vi "COB send.vi"(4 "Data":u8[](array[numeric]), 5 "error in (no error)":errorcluster, 7 "COB id":i32) -> (0 "error out":errorcluster)   [LabVIEW 2023, in "canopen.lvlib" / "CANopen.lvclass"]
doc: "Sends a bunch of data to a specific COB-ID."
uses:
  CANopen.lvclass
  <vilib>/xnet/xnet.llb/XNET Frame CAN.ctl
  <vilib>/xnet/xnet.llb/XNET Frame Type CAN.ctl
  <vilib>/xnet/xnet.llb/XNET Write (Frame CAN).vi
panel:
  out "session out":refnum<k21>
  in  "session in":refnum<k21>
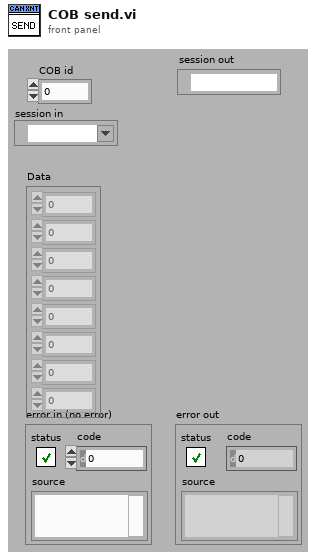
[diagram p1: front panel]
types:
  T1 = typedef "XNET Frame CAN.ctl" = cluster{"timestamp":timestamp, "payload":u8[], "identifier":u32, "type":T2, "extended?":bool, "echo?":bool}
  T2 = typedef "XNET Frame Type CAN.ctl" = u8
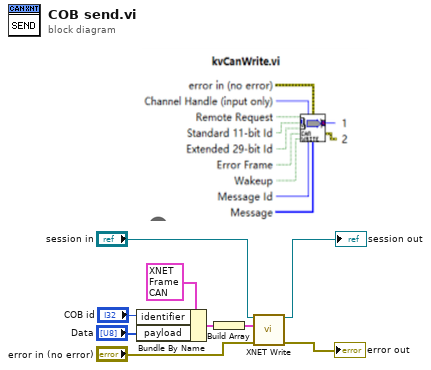
[diagram p0: block diagram]
diagram:
  n1 = Bundle By Name(cluster=T1 {"timestamp"=timestamp(0 s since 1904-01-01), "payload"=[], "identifier"=0, "type"=0, "extended?"=FALSE, "echo?"=FALSE} ("CAN frame"), "identifier"="COB id", "payload"="Data") -> (w2:T1)
  n2 = Build Array(w2) -> (w1:T1[])
  n3 = call-poly <vilib>:"XNET Write.vi"("session in"="session in", "data"=w1, "error in (no error)"="error in (no error)") -> ("session out"=→"session out":refnum<k21>, "error out"=→"error out":errorcluster)  [unwired: 11 in]
